vi "Windows UI.vi"() -> ()   [LabVIEW 2015]
doc: "This is the primary Host VI."
panel:
  in  "IP Address":string="192.168.8.212"
  out "Display Battery State":bool
  out "Current Temperature":dbl(knob) scale=20.0..40.0
  out "Battery State":enum16{"Charged", "Running", "Low Batt"}(ring)
  out "Display RPM":bool
  out "Display Temperature":bool
  out "Display Voltage":bool
  out "Temperature Warning":bool
  out "Current RPM":dbl(knob) scale=0.0..1000.0
  in  "Stop Button":bool
  out "Error Out":errorcluster
  out "Current Voltage":dbl(knob) scale=0.0..4.0
  out "Variable History":cluster{dbl, dbl, dbl}(graph)
  # "NOTE: Update with your eval device IP address and select Edit>>Make Current Values Default before running"
  # "LCD Controls"
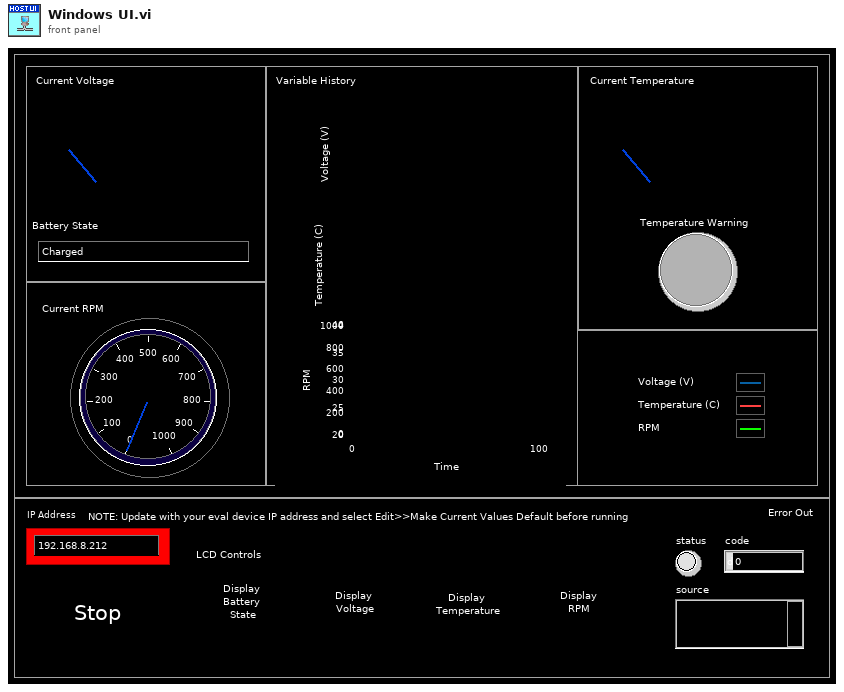
[diagram p1: front panel]
types:
  T1 = cluster{"Temperature Ref":refnum<k21>, "Temperature Warning Ref":refnum<k21>, "Voltage Ref":refnum<k21>, "Battery State Ref":refnum<k21>, "RPM Ref":refnum<k21>, "Display State Ref":refnum<k21>}
  T2 = typedef "Display State.ctl" = enum16{"Battery State", "RPM", "Temp", "Voltage"}
  T3 = cluster{"Temperature":fxp<+/-,32,13>, "Temperature Warning":bool, "Voltage":fxp<+/-,24,5>, "Battery State":enum16{"Charged", "Running", "Low Batt"}, "RPM":fxp<+,32,16>, "Display State":T2}
  T4 = cluster{"Voltage":fxp<+/-,24,5>, "Temperature":fxp<+/-,32,13>, "RPM":fxp<+,32,16>}
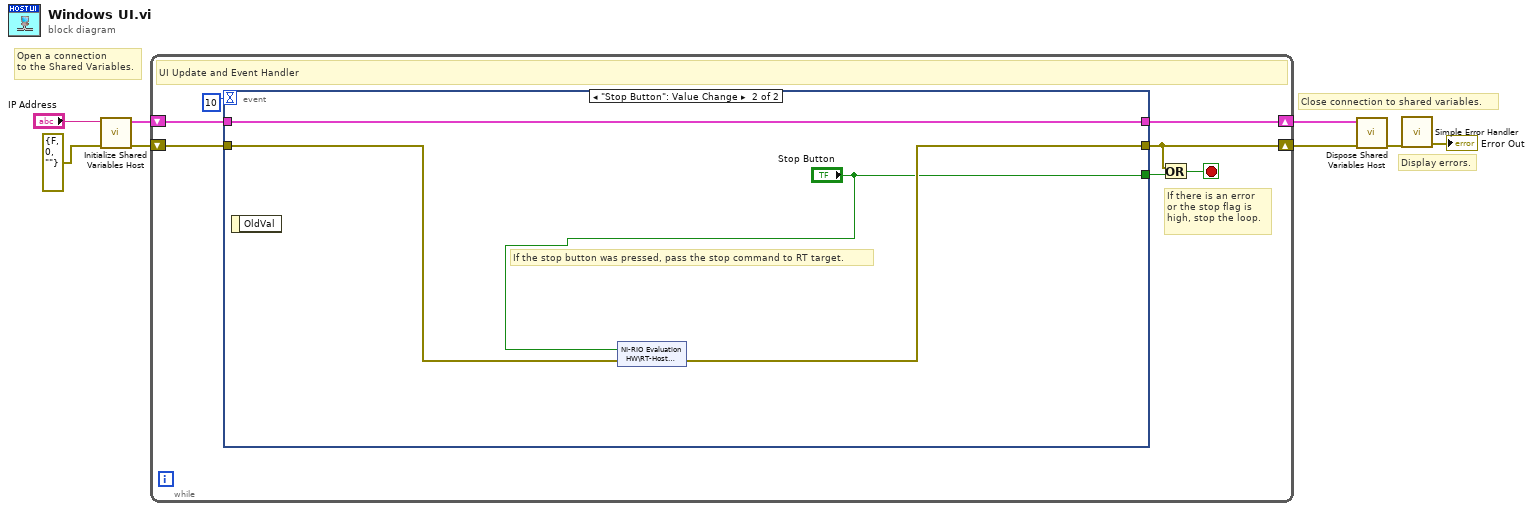
[diagram p0: block diagram]
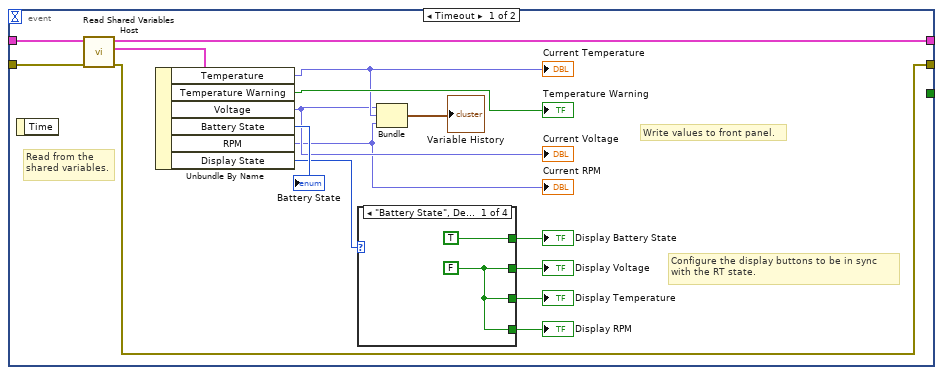
[diagram p2: hidden frame]
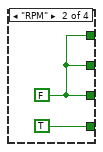
[diagram p3: hidden frame]
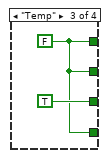
[diagram p4: hidden frame]
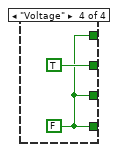
[diagram p5: hidden frame]
diagram:
  # "Close connection to shared variables."
  # "Display errors."
  # "Open a connection\nto the Shared Variables."
  n1 = call "Initialize Shared Variables Host.vi"("error in (no error)"=errorcluster {"status"=FALSE, "code"=0, "source"=""} ("error out"), "IP Address (No Slashes)"="IP Address") -> ("error out"=w7:errorcluster, "Shared Variable References"=w8:T1)  [unwired: 8 in]
  n2 = while {
    shift-right: [w10] -> w5
    shift-left: w7 -> [w15]
    shift-right: [w12] -> w6
    shift-left: w8 -> [w13]
    stop <- w11 stop-if-true
    # "UI Update and Event Handler"
    # "If there is an error\nor the stop flag is \nhigh, stop the loop."
    n3 = event shown="[1] \"Stop Button\": Value Change" {
      selector: _ -> [_ _]
      dyn-events: _ -> [_ _]
      timeout: 10 -> [_ _]
      tunnel: [w29 w41] -> w10
      tunnel: w15 -> [w30 w42]
      tunnel: w13 -> [w31 w43]
      tunnel: [w24 w43] -> w12
      tunnel: [_ "Stop Button"] -> w9
      event Timeout {
        # "Write values to front panel."
        # "Read from the\nshared variables."
        # "Configure the display buttons to be in sync\nwith the RT state."
        n4 = event-data() -> ()  [unwired: 1 in, 1 out]
        n5 = call "Read Shared Variables Host.vi"("error in (no error)"=w30, "Shared Variable References"=w31) -> ("error out"=w29:errorcluster, "Current Values"=w23:T3, "Shared Variable References Out"=w24:T1)  [unwired: 7 in]
        n6 = Unbundle By Name(w23) -> ("Temperature"=w18:fxp<+/-,32,13>, "Temperature Warning"=→"Temperature Warning":bool, "Voltage"=w17:fxp<+/-,24,5>, "Battery State"=→"Battery State":enum16{"Charged", "Running", "Low Batt"}, "RPM"=w16:fxp<+,32,16>, "Display State"=w20:T2)
        "Current Voltage" <- w17
        "Current RPM" <- w16
        "Current Temperature" <- w18
        n7 = case shown="\"Battery State\", Default" w20 {
          tunnel: [TRUE ("Display Battery State") w34 w36 w38] -> w28
          tunnel: [w32 w34 w36 TRUE ("Display Battery State")] -> w27
          tunnel: [w32 w34 TRUE ("Display Battery State") w38] -> w26
          tunnel: [w32 TRUE ("Display Battery State") w36 w38] -> w25
          frame "Battery State", Default {
            w32 = FALSE
          }
          frame "RPM" {
            w34 = FALSE
          }
          frame "Temp" {
            w36 = FALSE
          }
          frame "Voltage" {
            w38 = FALSE
          }
        }
        "Display Battery State" <- w28
        "Display Voltage" <- w27
        "Display Temperature" <- w26
        "Display RPM" <- w25
        n8 = Bundle("Voltage"=w17, "Temperature"=w18, "RPM"=w16) -> (→"Variable History":T4)  [unwired: 1 in]
      }
      event "Stop Button": Value Change {
        # "If the stop button was pressed, pass the stop command to RT target."
        n9 = event-data() -> ()  [unwired: 1 in, 1 out]
        n10 = shared-variable "NI-RIO Evaluation HW\\RT-Host Shared Variables.lvlib\\Stop"("Stop Button", error in=w42) -> (error out=w41:errorcluster)
      }
    }
    n11 = Or(x=w10, y=w9) -> (x .or. y?=w11:bool)
  }
  n12 = call "Dispose Shared Variables Host.vi"("error in (no error)"=w5, "Shared Variable References"=w6) -> ("error out"=w2:errorcluster)  [unwired: 9 in]
  n13 = call <vilib>:"Simple Error Handler.vi"("error in (no error)"=w2) -> ("error out"=→"Error Out":errorcluster)  [unwired: 4 in, 4 out]
